vi "Git Flow Delete.vi"(8 "error in (no error)":errorcluster, 11 "Git in":refnum<class "Git.lvclass">) -> (0 "error out":errorcluster, 2 "standard output":string, 3 "Git out":refnum<class "Git.lvclass">)   [LabVIEW 2019, in "Git.lvclass"]
uses:
  Git.lvclass
  Typedefs/Commands.git-flow--combo.ctl
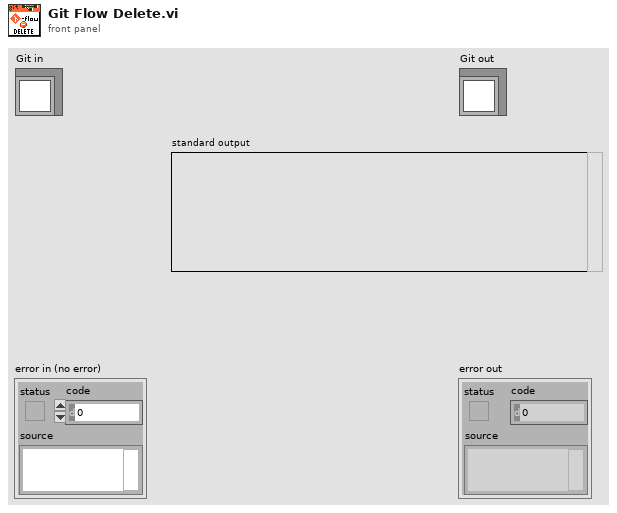
[diagram p1: front panel]
types:
  T1 = typedef "Git.lvclass/Commands.git-flow--combo.ctl" = string
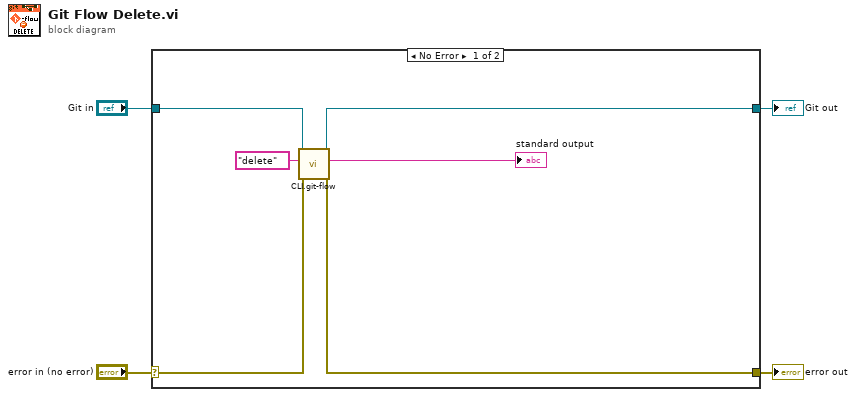
[diagram p0: block diagram]
diagram:
  n1 = case shown="No Error" "error in (no error)" {
    selector: "error in (no error)" -> [w10 w12]
    tunnel: [w9 w12] -> w3
    tunnel: [w8 w11] -> w1
    tunnel: "Git in" -> [w7 w11]
    frame No Error {
      n2 = call "CLI.git-flow.vi"("error in (no error)"=w10, "Command"=T1 "delete", "Git in"=w7) -> ("error out"=w9:errorcluster, "standard output"=→"standard output":string, "Git out"=w8:refnum<class "Git.lvclass">)  [unwired: 4 in, 2 out]
    }
    frame Error {
    }
  }
  "error out" <- w3
  "Git out" <- w1
